vi "readFilterData.vi"() -> ()   [LabVIEW 2026]
uses:
  <vilib>/Utility/miscctls.llb/LVRectTypeDef.ctl
  <vilib>/Utility/miscctls.llb/LVPointTypeDef.ctl
  <userlib>/Sensor.ctl
  <vilib>/measure/maspectr.llb/FFT Spectrum (Mag-Phase) for N Chan.vi
  <vilib>/Analysis/3filter.llb/Butterworth Filter (DBL).vi
  <vilib>/Instr/_visa.llb/VISA Configure Serial Port (Instr).vi
  <vilib>/measure/NI_MAPro.lvlib
  <vilib>/Analysis/NI_AALBase.lvlib
panel:
  in  "Time Target (s)":dbl=60.0
  out "SyncStop 2":bool
  out "Result":dbl
  in  "UvodniStranka":bool
  in  "ExitApp":bool
  in  "error in (no error)":errorcluster
  in  "Tab Control":T1(tab)
  in  "Playground":bool
  in  "UlohaACC":bool
  in  "UlohaEDA":bool
  in  "UlohaEEG":bool
  in  "UlohaEMG":bool
  in  "UlohaEKG":bool
  in  "StartMeasureEKG":bool
  in  "StopMeasureEKG":bool
  in  "HintEKG":bool
  out "GraphEKG":waveform(dbl)[](graph)
  out "ChartEKG":dbl(graph)
  in  "Vstupní COM port 2":refnum<visa-resource-name>
  out "BPM":i32
  out "size(s)":i32
  in  "Doba mìøení (s)":dbl=1.0 caption="Time Target (s)"
  out "SpectrumPlayground":cluster{"f0":dbl, "df":dbl, "magnitude":dbl[]}[](graph)
  in  "Filtr":bool
  in  "SaveFileButton":bool
  out "Waveform Graph":waveform(dbl)[](graph)
  in  "Horní mezní frekvence":dbl=0.45000000000000007 format="%0.2f"
  in  "Dolní mezní frekvence":dbl=0.12500000000000006 format="%0.4f"
  in  "Typ filtru":T2(ring)
  in  "OdstranitFiltr":bool
  in  "DeleteSignal":bool
  out "Waveform Chart":dbl(graph)
  in  "SendToFilter":bool
  out "Waveform":waveform(dbl)(graph)
  out "SyncStop":bool
  in  "Vstupní COM port":refnum<visa-resource-name>
  in  "Vzorkovací frekvence (Hz)":enum16{"1", "10", "100", "1000"}(ring)
  in  "Druh signálu":T3
  in  "StartMeasure":bool
  in  "StopMeasure":bool
  in  "Radio Buttons":T4(radio)
  # "Aplikace pro mìøení na platformì PLUX BITalino"
  # "EKG"
  # "Vstupní COM port"
  # "EEG"
  # "EDA"
  # "ACC"
  # "EMG"
  # "A1"
  # "A2"
  # "A3"
  # "A4"
  # "A5"
  # "A6"
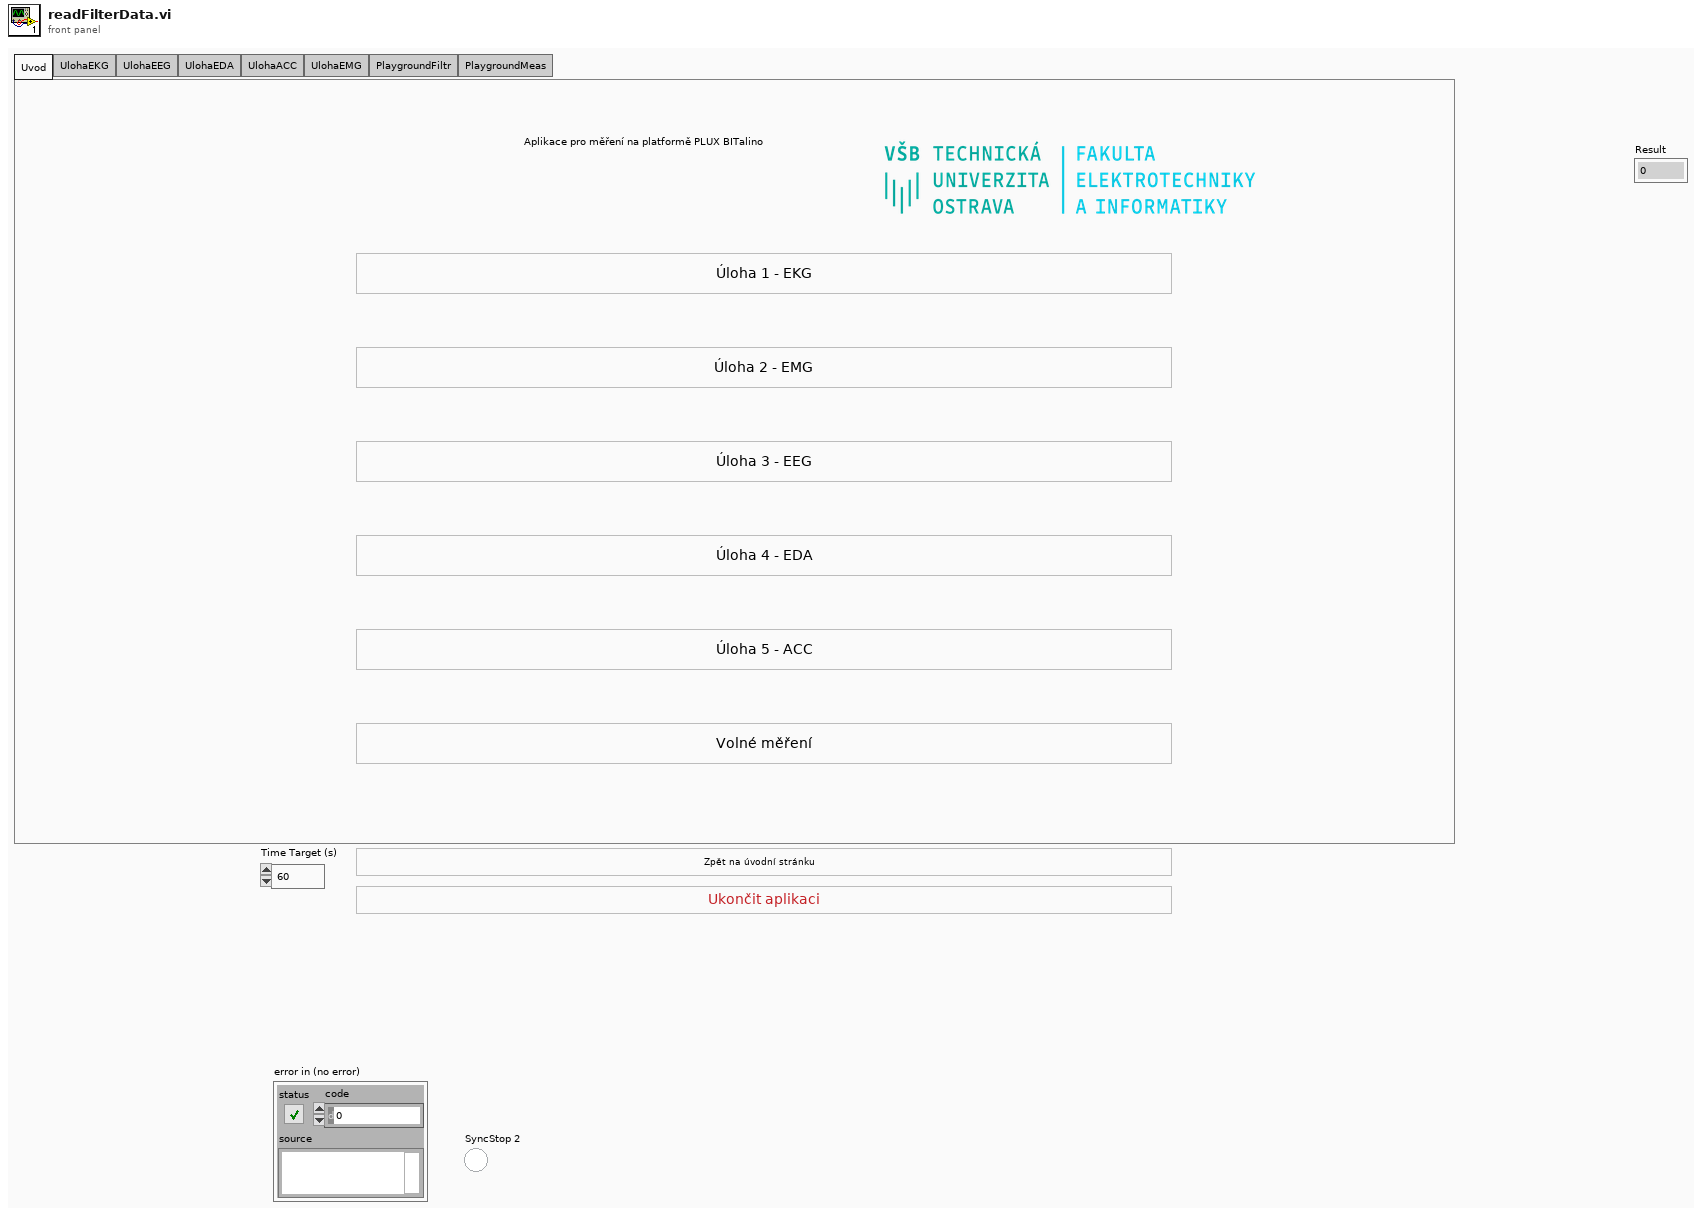
[diagram p1: front panel]
types:
  T1 = enum32{"Uvod", "UlohaEKG", "UlohaEEG", "UlohaEDA", "UlohaACC", "UlohaEMG", "PlaygroundFiltr", "PlaygroundMeas"}
  T2 = enum32{"Lowpass", "Highpass", "Bandpass", "Bandstop"}
  T3 = cluster{"Signál na kanálu A1":enum16{"EMG", "ECG", "EEG", "EDA", "ACC"}, "Signál na kanálu A2":enum16{"EMG", "ECG", "EEG", "EDA", "ACC"}, "Signál na kanálu A3":enum16{"EMG", "ECG", "EEG", "EDA", "ACC"}, "Signál na kanálu A4":enum16{"EMG", "ECG", "EEG", "EDA", "ACC"}, "Signál na kanálu A5":enum16{"EMG", "ECG", "EEG", "EDA", "ACC"}, "Signál na kanálu A6":enum16{"EMG", "ECG", "EEG", "EDA", "ACC"}}
  T4 = enum32{"Item 0", "Item 1", "Item 2", "Item 3", "Item 4", "Item 5"}
  T5 = enum16{"Wait", "Exit", "Measure", "Intro", "UlohaEKG", "UlohaEMG", "PlaygroundMeas", "UlohaEEG", "UlohaEDA", "UlohaACC", "PlaygroundFiltr", "SaveFile", "FilterSignal", "RemoveFilter", "HintEKG", "DeleteSignal"}
  T6 = enum16{"Always On", "Always Off", "Off While Running"}
  T7 = enum32{"Uvod", "UlohaEKG", "UlohaEEG", "UlohaEDA", "UlohaACC", "UlohaEMG", "PlaygroundFiltr"}
  T8 = typedef "LVPointTypeDef.ctl" = cluster{"Horizontal":i16, "Vertical":i16}
  T9 = typedef "LVRectTypeDef.ctl" = cluster{"Left":i16, "Top":i16, "Right":i16, "Bottom":i16}
  T10 = enum8{"Enabled", "Disabled", "Disabled and Grayed Out"}
  T11 = typedef "Sensor.ctl" = enum16{"EMG", "ECG", "EEG", "EDA", "ACC", "LUX"}
  T12 = cluster{"Sensor 1":T11, "Sensor 2":T11, "Sensor 3":T11, "Sensor 4":T11, "Sensor 5":T11, "Sensor 6":T11}
  T13 = cluster{"Result":dbl, "Result":dbl, "Result":dbl, "Result":dbl, "Result":dbl, "Result":dbl}
  T14 = enum16{"Wait", "Exit", "Measure", "Intro", "UlohaEKG", "UlohaEMG", "PlaygroundMeas", "UlohaEEG", "UlohaEDA", "UlohaACC", "PlaygroundFiltr", "SaveFile", "FilterSignal", "RemoveFilter", "HintEKG"}
  T15 = enum16{"Wait", "Exit", "Measure", "Intro", "UlohaEKG", "UlohaEMG", "PlaygroundMeas", "UlohaEEG", "UlohaEDA", "UlohaACC"}
  T16 = enum16{"Wait", "Exit", "Measure", "Intro", "UlohaEKG", "UlohaEMG", "PlaygroundMeas"}
  T17 = enum16{"Wait", "Exit", "Measure", "Intro", "UlohaEKG", "UlohaEMG"}
  T18 = enum16{"Wait", "Exit", "Measure", "Intro", "UlohaEKG", "UlohaEMG", "PlaygroundMeas", "UlohaEEG", "UlohaEDA", "UlohaACC", "PlaygroundFiltr"}
  T19 = enum16{"Wait", "Exit", "Measure", "Intro", "UlohaEKG", "UlohaEMG", "PlaygroundMeas", "UlohaEEG", "UlohaEDA", "UlohaACC", "PlaygroundFiltr", "SaveFile"}
  T20 = enum16{"Wait", "Exit", "Measure", "Intro", "UlohaEKG", "UlohaEMG", "PlaygroundMeas", "UlohaEEG", "UlohaEDA", "UlohaACC", "PlaygroundFiltr", "SaveFile", "FilterSignal", "RemoveFilter"}
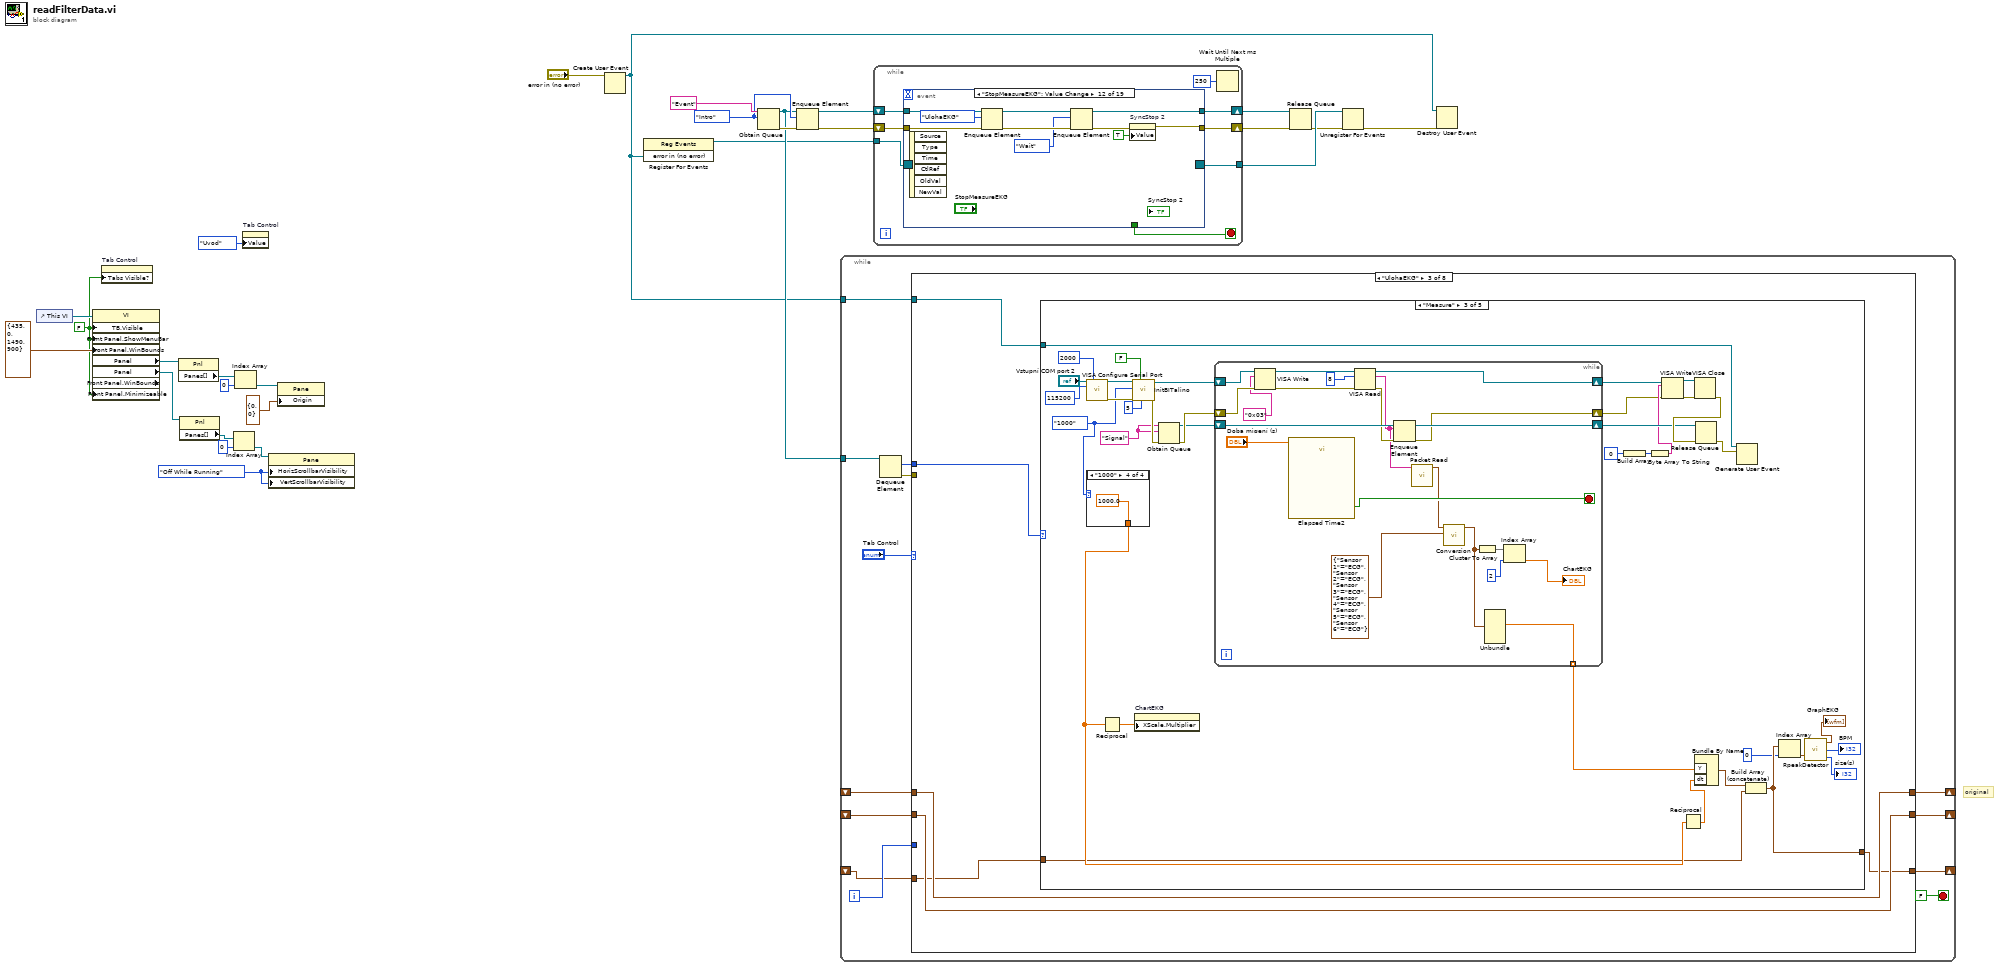
[diagram p0: block diagram]
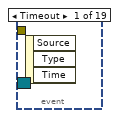
[diagram p2: hidden frame]
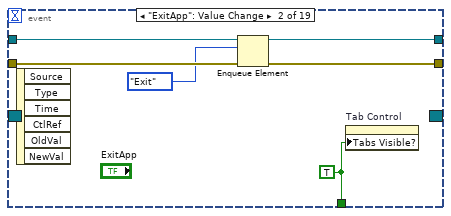
[diagram p3: hidden frame]
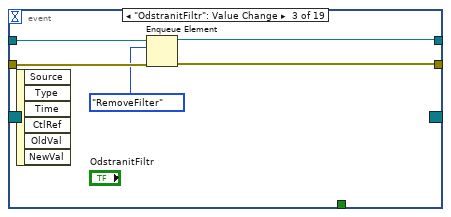
[diagram p4: hidden frame]
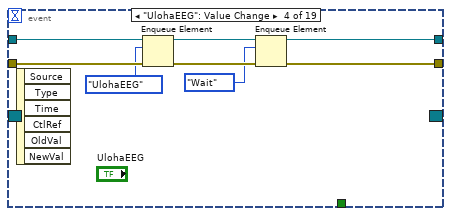
[diagram p5: hidden frame]
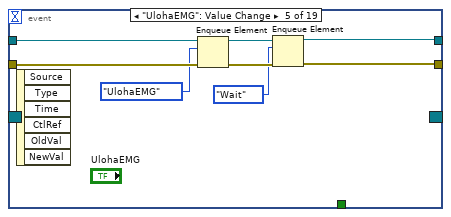
[diagram p6: hidden frame]
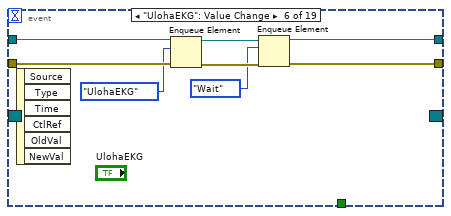
[diagram p7: hidden frame]
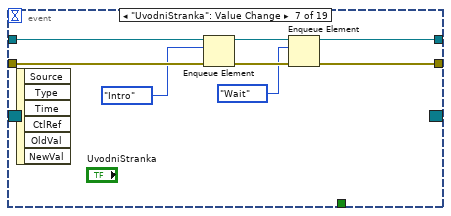
[diagram p8: hidden frame]
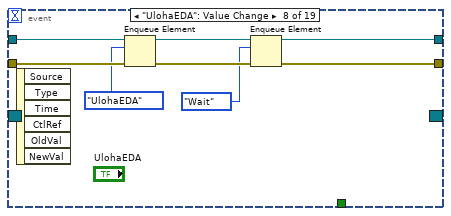
[diagram p9: hidden frame]
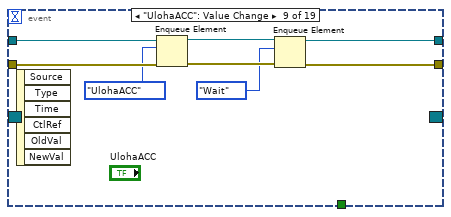
[diagram p10: hidden frame]
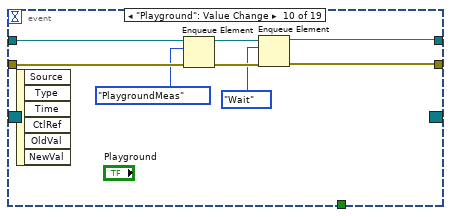
[diagram p11: hidden frame]
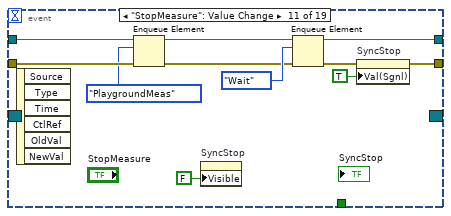
[diagram p12: hidden frame]
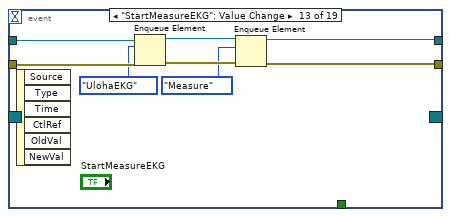
[diagram p13: hidden frame]
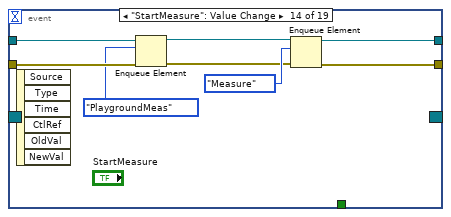
[diagram p14: hidden frame]
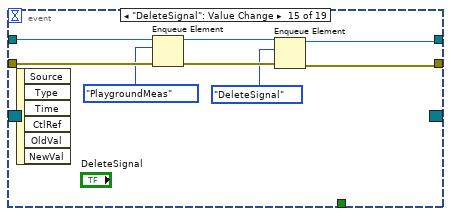
[diagram p15: hidden frame]
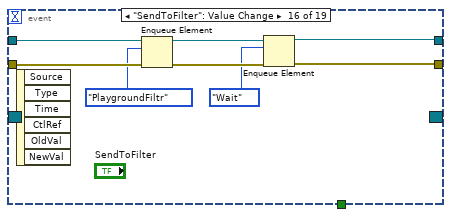
[diagram p16: hidden frame]
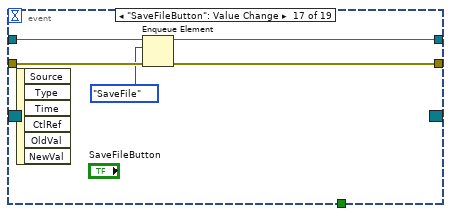
[diagram p17: hidden frame]
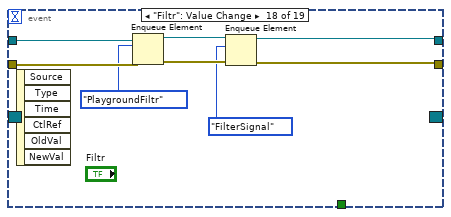
[diagram p18: hidden frame]
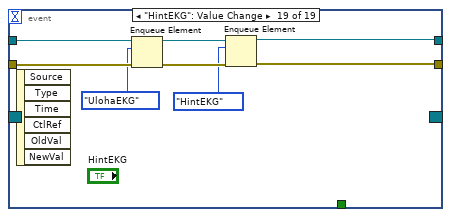
[diagram p19: hidden frame]
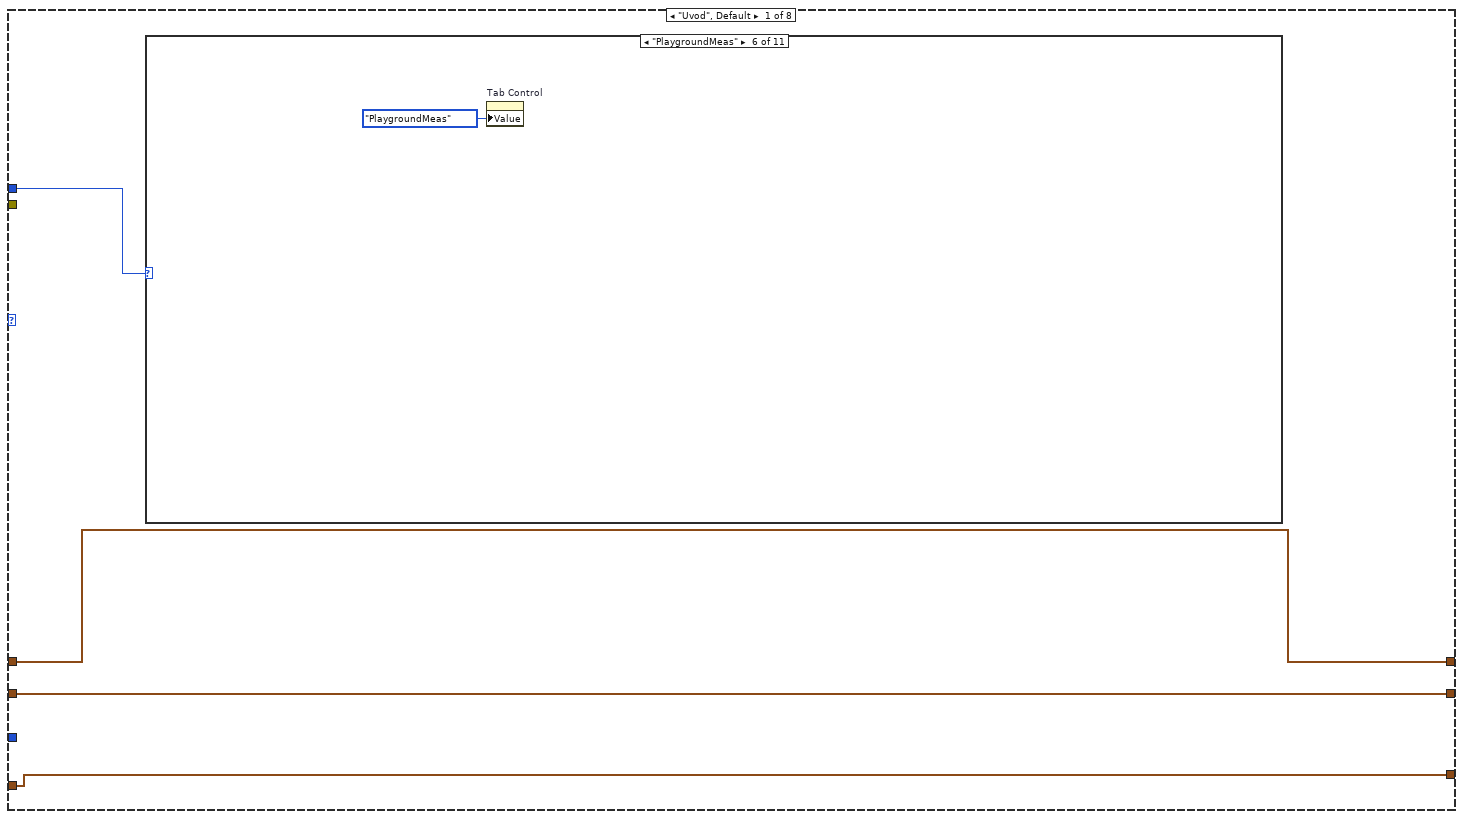
[diagram p20: hidden frame]
diagram:
  w10 = T5."Intro"
  w16 = T6."Off While Running" ("Horizontal Scrollbar Visibility")
  w15 = FALSE ("Front Panel Window:Closeable")
  # "original"
  n1 = control-ref of="This VI"() -> (w28:refnum<vi>)
  n2 = property class="VI" props=["TB.Visible", "Front Panel.ShowMenuBar", "Front Panel.WinBounds", "Panel", "Panel", "Front Panel.WinBounds", "Front Panel.Minimizeable"](reference=w28, "TB.Visible"=w15, "Front Panel.ShowMenuBar"=w15, "Front Panel.WinBounds"=T9 {"Left"=435, "Top"=0, "Right"=1490, "Bottom"=900} ("Front Panel Window:Window Bounds"), "Front Panel.Minimizeable"=w15) -> ("Panel"=w26:refnum<vi>, "Panel"=w20:refnum<vi>)  [unwired: 1 in, 3 out]
  n3 = property on="Tab Control" class="TabCtl (strict)"("Tabs Visible?"=w15) -> ()  [unwired: 2 in, 2 out]
  n4 = property class="Pnl"(reference=w26) -> ("Panes[]"=w25:refnum<vi>[])  [unwired: 1 in, 2 out]
  n5 = property class="Pnl"(reference=w20) -> ("Panes[]"=w19:refnum<vi>[])  [unwired: 1 in, 2 out]
  n6 = Index Array(array=w19, index=0) -> (element=w17:refnum<vi>)
  n7 = Index Array(array=w25, index=0) -> (element=w23:refnum<vi>)
  n8 = property on="Tab Control" class="TabCtl (strict)"("Value"=T7."Uvod" ("Tab Control")) -> ()  [unwired: 2 in, 2 out]
  n9 = property class="Pane"(reference=w17, "HorizScrollbarVisibility"=w16, "VertScrollbarVisibility"=w16) -> ()  [unwired: 1 in, 2 out]
  n10 = property class="Pane"(reference=w23, "Origin"=T8 {"Horizontal"=0, "Vertical"=0}) -> ()  [unwired: 1 in, 2 out]
  n11 = Create User Event(user event datatype="error in (no error)") -> (user event=w2:refnum<user-event>)  [unwired: 1 in, 1 out]
  n12 = register-events(w2) -> (reference out=w1:refnum<event-registration>)  [unwired: 2 in, 1 out]
  n13 = Obtain Queue(name (unnamed)="Event", element data type=w10) -> (queue out=w9:refnum<queue>, error out=w13:errorcluster)  [unwired: 3 in, 1 out]
  n14 = Enqueue Element(queue=w9, element=w10, error in (no error)=w13) -> (queue out=w12:refnum<queue>, error out=w11:errorcluster)  [unwired: 1 in, 1 out]
  n15 = while {
    shift-right: [w41] -> _
    shift-left: _ -> [w33]
    tunnel: w9 -> [w37]
    tunnel: w2 -> [w36]
    shift-right: [w32] -> _
    shift-left: _ -> [w31]
    shift-right: [w30] -> _
    shift-left: _ -> [w29]
    i -> [w40]
    stop <- FALSE stop-if-true
    n16 = Dequeue Element(queue=w37) -> (element=w38:T5, error out=w35:errorcluster)  [unwired: 2 in, 2 out]
    n17 = case shown="\"UlohaEKG\"" "Tab Control" {
      tunnel: [w45 w60 w96 w172 w180 w188 w196 w204] -> w41
      tunnel: w33 -> [w45 w61 w96 w172 w180 w188 w196 w203]
      tunnel: w40 -> [_ _ _ _ _ _ _ _]
      tunnel: w38 -> [w44 w62 w99 w171 w179 w187 w195 w207]
      tunnel: w36 -> [_ _ w98 _ _ _ _ w206]
      tunnel: w35 -> [_ _ _ _ _ _ _ w205]
      tunnel: [w43 w59 w97 w170 w178 w186 w194 w202] -> w32
      tunnel: w31 -> [w43 w58 w97 w170 w178 w186 w194 w202]
      tunnel: [w42 w57 w95 w169 w177 w185 w193 w201] -> w30
      tunnel: w29 -> [w42 w57 w94 w169 w177 w185 w193 w201]
      frame "Uvod", Default {
        n18 = case shown="\"PlaygroundMeas\"" w44 {
          frame "Wait", Default {
            n19 = property on="UvodniStranka" class="Bool"("DisabledEnum"=T10."Disabled and Grayed Out" ("Disabled")) -> ()  [unwired: 2 in, 2 out]
            n20 = property on="Tab Control" class="TabCtl (strict)"("Tabs Visible?"=FALSE) -> ()  [unwired: 2 in, 2 out]
          }
          frame "UlohaEKG" {
            n21 = property on="Tab Control" class="TabCtl (strict)"("Value"=T1."UlohaEKG" ("Tab Control")) -> ()  [unwired: 2 in, 2 out]
          }
          frame "UlohaEMG" {
            n22 = property on="Tab Control" class="TabCtl (strict)"("Value"=T1."UlohaEMG" ("Tab Control")) -> ()  [unwired: 2 in, 2 out]
          }
          frame "Exit" {
            n23 = flat-sequence {
              frame #0 {
                n24 = property on="Tab Control" class="TabCtl (strict)"("Value"=T1."Uvod" ("Tab Control")) -> ()  [unwired: 2 in, 2 out]
              }
              frame #1 {
                n25 = Stop(stop? (T)=TRUE) -> ()
              }
            }
          }
          frame "Intro" {
            n26 = property on="Tab Control" class="TabCtl (strict)"("Value"=T1."Uvod" ("Tab Control")) -> ()  [unwired: 2 in, 2 out]
          }
          frame "PlaygroundMeas" {
            n27 = property on="Tab Control" class="TabCtl (strict)"("Value"=T1."PlaygroundMeas" ("Tab Control")) -> ()  [unwired: 2 in, 2 out]
          }
          frame "Measure" {
          }
          frame "UlohaEEG" {
            n28 = property on="Tab Control" class="TabCtl (strict)"("Value"=T1."UlohaEEG" ("Tab Control")) -> ()  [unwired: 2 in, 2 out]
          }
          frame "UlohaEDA" {
            n29 = property on="Tab Control" class="TabCtl (strict)"("Value"=T1."UlohaEDA" ("Tab Control")) -> ()  [unwired: 2 in, 2 out]
          }
          frame "UlohaACC" {
            n30 = property on="Tab Control" class="TabCtl (strict)"("Value"=T1."UlohaACC" ("Tab Control")) -> ()  [unwired: 2 in, 2 out]
          }
          frame "PlaygroundFiltr" {
          }
        }
      }
      frame "PlaygroundFiltr" {
        n31 = case shown="\"RemoveFilter\"" w62 {
          tunnel: w61 -> [w64 w71 w82 w84 w88 w92]
          tunnel: [w64 w69 w82 w84 w88 w92] -> w60
          tunnel: [w64 w69 w79 w83 w87 w91] -> w59
          tunnel: w58 -> [_ w68 w79 w83 w87 w91]
          frame "Wait", Default {
            n32 = property on="UvodniStranka" class="Bool"("DisabledEnum"=T10."Enabled" ("Disabled")) -> ()  [unwired: 2 in, 2 out]
            n33 = Build Array(w64) -> (w63:waveform(dbl)[])
            "Waveform Graph" <- w63
            n34 = call-poly <vilib>:"FFT Spectrum (Mag-Phase).vi"("time signals"=w63) -> ("magnitudes"=w65:cluster{"f0":dbl, "df":dbl, "magnitude":dbl[]}[])  [unwired: 6 in, 4 out]
            n35 = local write "SpectrumPlayground"(w65) -> ()
          }
          frame "FilterSignal" {
            n36 = Unbundle By Name(w71) -> ("Y"=w73:dbl[], "dt"=w70:dbl)
            n37 = Reciprocal(x=w70) -> (1/x=w72:dbl)
            n38 = call-poly <vilib>:"Butterworth Filter.vi"("filter type"="Typ filtru", "low cutoff freq: fl"="Dolní mezní frekvence", "high cutoff freq: fh"="Horní mezní frekvence", "sampling freq: fs"=w72, "X"=w73) -> ("Filtered X"=w74:dbl[])  [unwired: 3 in, 1 out]
            n39 = Bundle By Name("Y"=w74, "dt"=w70) -> (w69:waveform(dbl))  [unwired: 1 in]
            n40 = Build Array(w68, w69) -> (w67:waveform(dbl)[])
            n41 = call-poly <vilib>:"FFT Spectrum (Mag-Phase).vi"("time signals"=w67) -> ("magnitudes"=→"SpectrumPlayground":cluster{"f0":dbl, "df":dbl, "magnitude":dbl[]}[])  [unwired: 6 in, 4 out]
            n42 = local write "Waveform Graph"(w67) -> ()
          }
          frame "RemoveFilter" {
            n43 = Build Array(w79, w79) -> (w80:waveform(dbl)[])
            n44 = local write "Waveform Graph"(w80) -> ()
            n45 = call-poly <vilib>:"FFT Spectrum (Mag-Phase).vi"("time signals"=w80) -> ("magnitudes"=w81:cluster{"f0":dbl, "df":dbl, "magnitude":dbl[]}[])  [unwired: 6 in, 4 out]
            n46 = local write "SpectrumPlayground"(w81) -> ()
          }
          frame "Exit" {
            n47 = flat-sequence {
              frame #0 {
                n48 = property on="Tab Control" class="TabCtl (strict)"("Value"=T1."Uvod" ("Tab Control")) -> ()  [unwired: 2 in, 2 out]
              }
              frame #1 {
                n49 = Stop(stop? (T)=TRUE) -> ()
              }
            }
          }
          frame "Intro" {
            n50 = property on="Tab Control" class="TabCtl (strict)"("Value"=T1."Uvod" ("Tab Control")) -> ()  [unwired: 2 in, 2 out]
          }
          frame "SaveFile" {
            n51 = local read "Waveform"() -> (w93:waveform(dbl))
            n52 = call "saveFile(subVI).vi"("Typ signálu"="EMG", "Vstupní signál"=w93) -> ()  [unwired: 1 in]
          }
        }
      }
      frame "UlohaEKG" {
        n53 = case shown="\"Measure\"" w99 {
          tunnel: w98 -> [_ _ w120 _ _]
          tunnel: [w100 w102 w112 w166 w167] -> w95
          tunnel: w94 -> [w100 w102 w113 w166 w167]
          frame "Wait", Default {
            n54 = property on="UvodniStranka" class="Bool"("DisabledEnum"=T10."Enabled" ("Disabled")) -> ()  [unwired: 2 in, 2 out]
          }
          frame "Exit" {
            n55 = flat-sequence {
              frame #0 {
                n56 = property on="Tab Control" class="TabCtl (strict)"("Value"=T1."Uvod" ("Tab Control")) -> ()  [unwired: 2 in, 2 out]
              }
              frame #1 {
                n57 = Stop(stop? (T)=TRUE) -> ()
              }
            }
          }
          frame "Measure" {
            w115 = enum16{"1", "10", "100", "1000"}."1000" ("Sample Rate")
            w122 = "Signal" ("name (unnamed)")
            n58 = call-poly "VISA Configure Serial Port"("VISA resource name"="Vstupní COM port 2", "timeout (10sec)"=u32 2000, "baud rate (9600)"=u32 115200) -> ("VISA resource name out"=w137:refnum<visa-resource-name>, "error out"=w136:errorcluster)  [unwired: 11 in]
            n59 = case shown="\"1000\"" w115 {
              tunnel: [1.0 10.0 100.0 1000.0] -> w116
              frame "1", Default {
              }
              frame "10" {
              }
              frame "100" {
              }
              frame "1000" {
              }
            }
            n60 = Reciprocal(x=w116) -> (1/x=w117:dbl)
            n61 = call "InitBITalino.vi"("Battery \nThreshold (%)"=u8 5 ("Battery \nThreshold (%)"), "MODE"=FALSE, "error in (no error)"=w136, "Sample Rate"=w115, "BITalino"=w137) -> ("error out"=w132:errorcluster, "VISA out"=w133:refnum<visa-resource-name>)  [unwired: 4 in, 1 out]
            n62 = property on="ChartEKG" class="WFChart (strict)"("XScale.Multiplier"=w117) -> ()  [unwired: 2 in, 2 out]
            n63 = Obtain Queue(name (unnamed)=w122, element data type=w122, error in (no error)=w132) -> (queue out=w119:refnum<queue>, error out=w131:errorcluster)  [unwired: 2 in, 1 out]
            n64 = while {
              shift-right: [w161] -> w130
              shift-left: w133 -> [w165]
              shift-right: [w157] -> w106
              shift-left: w131 -> [w164]
              shift-right: [w158] -> w126
              shift-left: w119 -> [w160]
              tunnel: [w146] -> w105 mode=indexing
              stop <- w156 stop-if-true
              n65 = VISA Write(VISA resource name=w165, write buffer="0x03", error in (no error)=w164) -> (VISA resource name out=w154:refnum<visa-resource-name>, error out=w162:errorcluster)  [unwired: 1 out]
              n66 = call "Elapsed Time2"("Time Target (s)"="Doba mìøení (s)") -> ("Time has Elapsed"=w156:bool)  [unwired: 11 in, 7 out]
              n67 = VISA Read(VISA resource name=w154, byte count=u32 8, error in (no error)=w162) -> (VISA resource name out=w161:refnum<visa-resource-name>, read buffer=w145:string, error out=w159:errorcluster)  [unwired: 1 out]
              n68 = Enqueue Element(queue=w160, element=w145, error in (no error)=w159) -> (queue out=w158:refnum<queue>, error out=w157:errorcluster)  [unwired: 1 in, 1 out]
              n69 = call "Packet Read.vi"("Packets"=w145) -> ("Analog Channels"=w147:cluster{u16, u16, u16, u16, u16, u16})  [unwired: 7 in, 3 out]
              n70 = call "Conversion.vi"("Sensor Type"=T12 {"Sensor 1"=enum."ECG", "Sensor 2"=enum."ECG", "Sensor 3"=enum."ECG", "Sensor 4"=enum."ECG", "Sensor 5"=enum."ECG", "Sensor 6"=enum."ECG"}, "Analog Channels"=w147) -> ("output cluster"=w148:T13)  [unwired: 8 in, 1 out]
              n71 = Cluster To Array(cluster=w148) -> (array=w151:dbl[])
              n72 = Unbundle(w148) -> ("Result"=w146:dbl)  [unwired: 5 out]
              n73 = Index Array(array=w151, index=2) -> (element=→"ChartEKG":dbl)
            }
            n74 = Build Array(u8 0) -> (w124:u8[])
            n75 = Byte Array To String(unsigned byte array=w124) -> (string=w123:string)
            n76 = VISA Write(VISA resource name=w130, write buffer=w123, error in (no error)=w106) -> (VISA resource name out=w129:refnum<visa-resource-name>, error out=w128:errorcluster)  [unwired: 1 out]
            n77 = Reciprocal(x=w116) -> (1/x=w118:dbl)
            n78 = VISA Close(VISA resource name=w129, error in (no error)=w128) -> (error out=w127:errorcluster)
            n79 = Bundle By Name("Y"=w105, "dt"=w118) -> (w114:waveform(dbl))  [unwired: 1 in]
            n80 = Release Queue(queue=w126, error in (no error)=w127) -> (error out=w121:errorcluster)  [unwired: 1 in, 2 out]
            n81 = Generate User Event(user event=w120, event data cluster=w121) -> ()  [unwired: 2 in, 2 out]
            n82 = Build Array (concatenate)(w114, w113) -> (w112:waveform(dbl)[])
            n83 = Index Array(array=w112, index=0) -> (element=w110:waveform(dbl))
            n84 = call "RpeakDetector.vi"("Vstupní signál"=w110) -> ("Signál s peaky"=→"GraphEKG":waveform(dbl)[], "BPM"=→"BPM":i32, "size(s)"=→"size(s)":i32)
          }
          frame "HintEKG" {
            n85 = call "NapovedaEKG(subVI).vi"() -> ()  [unwired: 1 in]
          }
          frame "Intro" {
            n86 = property on="Tab Control" class="TabCtl (strict)"("Value"=T1."Uvod" ("Tab Control")) -> ()  [unwired: 2 in, 2 out]
          }
        }
      }
      frame "UlohaEEG" {
        n87 = case shown="\"Exit\"" w171 {
          frame "Wait", Default {
            n88 = property on="UvodniStranka" class="Bool"("DisabledEnum"=T10."Enabled" ("Disabled")) -> ()  [unwired: 2 in, 2 out]
          }
          frame "Exit" {
            n89 = flat-sequence {
              frame #0 {
                n90 = property on="Tab Control" class="TabCtl (strict)"("Value"=T1."Uvod" ("Tab Control")) -> ()  [unwired: 2 in, 2 out]
              }
              frame #1 {
                n91 = Stop(stop? (T)=TRUE) -> ()
              }
            }
          }
          frame "Measure" {
          }
          frame "Intro" {
            n92 = property on="Tab Control" class="TabCtl (strict)"("Value"=T1."Uvod" ("Tab Control")) -> ()  [unwired: 2 in, 2 out]
          }
          frame "UlohaEKG" {
          }
          frame "UlohaEMG" {
          }
          frame "PlaygroundMeas" {
          }
          frame "UlohaEEG" {
          }
          frame "UlohaEDA" {
          }
          frame "UlohaACC" {
          }
        }
      }
      frame "UlohaEDA" {
        n93 = case shown="\"Wait\", Default" w179 {
          frame "Wait", Default {
            n94 = property on="UvodniStranka" class="Bool"("DisabledEnum"=T10."Enabled" ("Disabled")) -> ()  [unwired: 2 in, 2 out]
          }
          frame "Exit" {
            n95 = flat-sequence {
              frame #0 {
                n96 = property on="Tab Control" class="TabCtl (strict)"("Value"=T1."Uvod" ("Tab Control")) -> ()  [unwired: 2 in, 2 out]
              }
              frame #1 {
                n97 = Stop(stop? (T)=TRUE) -> ()
              }
            }
          }
          frame "Measure" {
          }
          frame "Intro" {
            n98 = property on="Tab Control" class="TabCtl (strict)"("Value"=T1."Uvod" ("Tab Control")) -> ()  [unwired: 2 in, 2 out]
          }
          frame "UlohaEKG" {
          }
          frame "UlohaEMG" {
          }
          frame "PlaygroundMeas" {
          }
          frame "UlohaEEG" {
          }
          frame "UlohaEDA" {
          }
          frame "UlohaACC" {
          }
        }
      }
      frame "UlohaACC" {
        n99 = case shown="\"Wait\", Default" w187 {
          frame "Wait", Default {
            n100 = property on="UvodniStranka" class="Bool"("DisabledEnum"=T10."Enabled" ("Disabled")) -> ()  [unwired: 2 in, 2 out]
          }
          frame "Exit" {
            n101 = flat-sequence {
              frame #0 {
                n102 = property on="Tab Control" class="TabCtl (strict)"("Value"=T1."Uvod" ("Tab Control")) -> ()  [unwired: 2 in, 2 out]
              }
              frame #1 {
                n103 = Stop(stop? (T)=TRUE) -> ()
              }
            }
          }
          frame "Measure" {
          }
          frame "Intro" {
            n104 = property on="Tab Control" class="TabCtl (strict)"("Value"=T1."Uvod" ("Tab Control")) -> ()  [unwired: 2 in, 2 out]
          }
          frame "UlohaEKG" {
          }
          frame "UlohaEMG" {
          }
          frame "PlaygroundMeas" {
          }
          frame "UlohaEEG" {
          }
          frame "UlohaEDA" {
          }
          frame "UlohaACC" {
          }
        }
      }
      frame "UlohaEMG" {
        n105 = case shown="\"Intro\"" w195 {
          frame "Wait", Default {
            n106 = property on="UvodniStranka" class="Bool"("DisabledEnum"=T10."Enabled" ("Disabled")) -> ()  [unwired: 2 in, 2 out]
          }
          frame "Exit" {
            n107 = flat-sequence {
              frame #0 {
                n108 = property on="Tab Control" class="TabCtl (strict)"("Value"=T1."Uvod" ("Tab Control")) -> ()  [unwired: 2 in, 2 out]
              }
              frame #1 {
                n109 = Stop(stop? (T)=TRUE) -> ()
              }
            }
          }
          frame "Measure" {
          }
          frame "Intro" {
            n110 = property on="Tab Control" class="TabCtl (strict)"("Value"=T1."Uvod" ("Tab Control")) -> ()  [unwired: 2 in, 2 out]
          }
          frame "UlohaEKG" {
          }
          frame "UlohaEMG" {
          }
          frame "PlaygroundMeas" {
          }
        }
      }
      frame "PlaygroundMeas" {
        n111 = case shown="No Error" w205 {
          tunnel: w207 -> [w212 _]
          tunnel: [FALSE TRUE] -> _
          tunnel: w206 -> [w210 _]
          tunnel: [w209 w320] -> w204
          tunnel: w203 -> [w208 w320]
          frame No Error {
            n112 = case shown="\"Measure\"" w212 {
              tunnel: w210 -> [_ _ _ _ w236 _]
              tunnel: [w213 w216 w222 w224 w228 w317] -> w209
              tunnel: w208 -> [w213 w216 w222 w224 _ w317]
              frame "Wait", Default {
                n113 = property on="UvodniStranka" class="Bool"("DisabledEnum"=T10."Enabled" ("Disabled")) -> ()  [unwired: 2 in, 2 out]
                n114 = property on="SyncStop" class="Bool (strict)"("Val(Sgnl)"=FALSE ("Value (Signaling)")) -> ()  [unwired: 2 in, 2 out]
              }
              frame "Exit" {
                n115 = flat-sequence {
                  frame #0 {
                    w218 = waveform(dbl) {"t0"=timestamp(0 s since 1904-01-01), "dt"=1.0, "Y"=[0.0]} ("Waveform")
                    n116 = property on="Tab Control" class="TabCtl (strict)"("Value"=T1."Uvod" ("Tab Control")) -> ()  [unwired: 2 in, 2 out]
                    n117 = Build Array(w218, w218) -> (w217:waveform(dbl)[])
                    n118 = call-poly <vilib>:"FFT Spectrum (Mag-Phase).vi"("time signals"=w217) -> ("magnitudes"=w219:cluster{"f0":dbl, "df":dbl, "magnitude":dbl[]}[])  [unwired: 6 in, 4 out]
                    n119 = local write "SpectrumPlayground"(w219) -> ()
                    n120 = property on="Waveform Graph" class="WFGraph (strict)"("Value"=w217) -> ()  [unwired: 2 in, 2 out]
                  }
                  frame #1 {
                    n121 = Stop(stop? (T)=TRUE) -> ()
                  }
                }
              }
              frame "PlaygroundFiltr" {
                n122 = property on="Tab Control" class="TabCtl (strict)"("Value"=T1."PlaygroundFiltr" ("Tab Control")) -> ()  [unwired: 2 in, 2 out]
              }
              frame "Intro" {
                n123 = flat-sequence {
                  frame #0 {
                    n124 = property on="Tab Control" class="TabCtl (strict)"("Value"=T1."Uvod" ("Tab Control")) -> ()  [unwired: 2 in, 2 out]
                  }
                  frame #1 {
                    n125 = Wait (ms)(milliseconds to wait=u32 100) -> ()  [unwired: 1 out]
                  }
                }
              }
              frame "Measure" {
                w238 = "Signal" ("name (unnamed)")
                n126 = property on="Vzorkovací frekvence (Hz)" class="Enum (strict)"() -> ("Value"=w231:enum16{"1", "10", "100", "1000"})  [unwired: 2 in, 2 out]
                n127 = call-poly "VISA Configure Serial Port"("VISA resource name"="Vstupní COM port", "timeout (10sec)"=u32 2000, "baud rate (9600)"=u32 115200) -> ("VISA resource name out"=w253:refnum<visa-resource-name>, "error out"=w252:errorcluster)  [unwired: 11 in]
                n128 = case shown="\"1000\"" w231 {
                  tunnel: [1.0 10.0 100.0 1000.0] -> w227
                  frame "1", Default {
                  }
                  frame "10" {
                  }
                  frame "100" {
                  }
                  frame "1000" {
                  }
                }
                n129 = Reciprocal(x=w227) -> (1/x=w230:dbl)
                n130 = call "InitBITalino.vi"("Battery \nThreshold (%)"=u8 5 ("Battery \nThreshold (%)"), "MODE"=FALSE, "error in (no error)"=w252, "Sample Rate"="Vzorkovací frekvence (Hz)", "BITalino"=w253) -> ("error out"=w248:errorcluster, "VISA out"=w249:refnum<visa-resource-name>)  [unwired: 4 in, 1 out]
                n131 = property on="Waveform Chart" class="WFChart (strict)"("XScale.Multiplier"=w230) -> ()  [unwired: 2 in, 2 out]
                n132 = Obtain Queue(name (unnamed)=w238, element data type=w238, error in (no error)=w248) -> (queue out=w237:refnum<queue>, error out=w247:errorcluster)  [unwired: 2 in, 1 out]
                n133 = while {
                  shift-right: [w310] -> w246
                  shift-left: w249 -> [w316]
                  shift-right: [w305] -> w229
                  shift-left: w247 -> [w315]
                  shift-right: [w306] -> w242
                  shift-left: w237 -> [w309]
                  stop <- w304 stop-if-true
                  n134 = VISA Write(VISA resource name=w316, write buffer="0x03", error in (no error)=w315) -> (VISA resource name out=w313:refnum<visa-resource-name>, error out=w312:errorcluster)  [unwired: 1 out]
                  n135 = call "Elapsed Time"("Time Target (s)"="Time Target (s)") -> ("Time has Elapsed"=w302:bool)  [unwired: 11 in, 7 out]
                  n136 = VISA Read(VISA resource name=w313, byte count=u32 8, error in (no error)=w312) -> (VISA resource name out=w310:refnum<visa-resource-name>, read buffer=w308:string, error out=w307:errorcluster)  [unwired: 1 out]
                  n137 = Enqueue Element(queue=w309, element=w308, error in (no error)=w307) -> (queue out=w306:refnum<queue>, error out=w305:errorcluster)  [unwired: 1 in, 1 out]
                  n138 = Unbundle By Name(w305) -> ("status"=w303:bool)
                  n139 = Or(x=w303, y=w302) -> (x .or. y?=w304:bool)
                }
                n140 = while {
                  tunnel: w237 -> [w266]
                  tunnel: [w262] -> w234 mode=indexing
                  tunnel: "Radio Buttons" -> [w261]
                  stop <- w263 stop-if-true
                  n141 = Dequeue Element(queue=w266) -> (element=w265:string, error out=w264:errorcluster)  [unwired: 2 in, 2 out]
                  n142 = case shown="No Error" w264 {
                    tunnel: w265 -> [w273 _]
                    tunnel: [FALSE TRUE] -> w263
                    tunnel: [w268 w299] -> w262
                    tunnel: w261 -> [w270 _]
                    frame No Error {
                      n143 = call "Packet Read.vi"("Packets"=w273) -> ("Analog Channels"=w272:cluster{u16, u16, u16, u16, u16, u16})  [unwired: 7 in, 3 out]
                      n144 = call "Conversion.vi"("Sensor Type"="Druh signálu", "Analog Channels"=w272) -> ("output cluster"=w269:T13)  [unwired: 8 in, 1 out]
                      n145 = case shown="\"Item 2\"" w270 {
                        tunnel: w269 -> [w277 w279 w284 w288 w292 w296]
                        tunnel: [w274 w278 w283 w287 w291 w295] -> w268
                        tunnel: "Druh signálu" -> [_ _ _ _ _ _]
                        frame "Item 0", Default {
                          n146 = Cluster To Array(cluster=w277) -> (array=w276:dbl[])
                          n147 = Index Array(array=w276, index=0) -> ()  [unwired: 1 out]
                          n148 = Unbundle(w277) -> ("Result"=w274:dbl)  [unwired: 5 out]
                        }
                        frame "Item 1" {
                          n149 = Cluster To Array(cluster=w279) -> (array=w281:dbl[])
                          n150 = Index Array(array=w281, index=1) -> ()  [unwired: 1 out]
                          n151 = Unbundle(w279) -> ("Result"=w278:dbl)  [unwired: 5 out]
                        }
                        frame "Item 2" {
                          n152 = Cluster To Array(cluster=w284) -> (array=w286:dbl[])
                          n153 = Unbundle(w284) -> ("Result"=w283:dbl)  [unwired: 5 out]
                          n154 = Index Array(array=w286, index=2) -> (element=→"Waveform Chart":dbl)
                        }
                        frame "Item 3" {
                          n155 = Cluster To Array(cluster=w288) -> (array=w290:dbl[])
                          n156 = Unbundle(w288) -> ("Result"=w287:dbl)  [unwired: 5 out]
                          n157 = Index Array(array=w290, index=3) -> ()  [unwired: 1 out]
                        }
                        frame "Item 4" {
                          n158 = Cluster To Array(cluster=w292) -> (array=w294:dbl[])
                          n159 = Unbundle(w292) -> ("Result"=w291:dbl)  [unwired: 5 out]
                          n160 = Index Array(array=w294, index=4) -> ()  [unwired: 1 out]
                        }
                        frame "Item 5" {
                          n161 = Cluster To Array(cluster=w296) -> (array=w298:dbl[])
                          n162 = Unbundle(w296) -> ("Result"=w295:dbl)  [unwired: 5 out]
                          n163 = Index Array(array=w298, index=5) -> ()  [unwired: 1 out]
                        }
                      }
                      "Result" <- w268
                    }
                    frame Error {
                      n164 = local read "Result"() -> (w299:dbl)
                    }
                  }
                }
                n165 = Build Array(u8 0) -> (w240:u8[])
                n166 = Byte Array To String(unsigned byte array=w240) -> (string=w239:string)
                n167 = VISA Write(VISA resource name=w246, write buffer=w239, error in (no error)=w229) -> (VISA resource name out=w245:refnum<visa-resource-name>, error out=w244:errorcluster)  [unwired: 1 out]
                n168 = VISA Close(VISA resource name=w245, error in (no error)=w244) -> (error out=w243:errorcluster)
                n169 = Release Queue(queue=w242, error in (no error)=w243) -> (error out=w235:errorcluster)  [unwired: 1 in, 2 out]
                n170 = Generate User Event(user event=w236, event data cluster=w235) -> ()  [unwired: 2 in, 2 out]
                n171 = Bundle By Name("Y"=w234, "dt"=w230) -> (w228:waveform(dbl))  [unwired: 1 in]
                "Waveform" <- w228
              }
              frame "DeleteSignal" {
                n172 = property on="Waveform Chart" class="WFChart (strict)"("History Data"=dbl[] []) -> ()  [unwired: 2 in, 2 out]
                n173 = local write "Waveform"(waveform(dbl) {"t0"=timestamp(0 s since 1904-01-01), "dt"=1.0, "Y"=[]} ("Waveform")) -> ()
              }
            }
          }
          frame Error {
          }
        }
      }
    }
  }
  n174 = while {
    shift-right: [w327] -> w7
    shift-left: w11 -> [w326]
    shift-right: [w328] -> w8
    shift-left: w12 -> [w329]
    tunnel: [w323] -> w5
    tunnel: w1 -> [w322]
    stop <- w325 stop-if-true
    n175 = event shown="[11] \"StopMeasureEKG\": Value Change" {
      selector: w322 -> [_ _ _ _ _ _ _ _ _ _ _ _ _ _ _ _ _ _ _]
      dyn-events: [_ _ _ _ _ _ _ _ _ _ _ _ _ _ _ _ _ _ _] -> w323
      timeout: _ -> [_ _ _ _ _ _ _ _ _ _ _ _ _ _ _ _ _ _ _]
      tunnel: w329 -> [_ w335 w340 w348 w356 w364 w372 w380 w388 w396 w401 w417 w425 w430 w441 w449 w454 w462 w470]
      tunnel: w326 -> [_ w334 w338 w347 w355 w363 w371 w379 w387 w395 w399 w416 w424 w428 w440 w448 w453 w459 w467]
      tunnel: [_ w333 w339 w344 w352 w360 w367 w377 w385 w390 w406 w413 w422 w433 w437 w445 w452 w460 w468] -> w328
      tunnel: [_ w332 w337 w342 w351 w358 w366 w376 w383 w392 w403 w409 w420 w432 w435 w443 w451 w457 w465] -> w327
      tunnel: [_ w330 _ _ _ _ _ _ _ _ _ _ _ _ _ _ _ _ _] -> w325
      event Timeout {
        n176 = event-data() -> ()  [unwired: 1 in, 3 out]
      }
      event "ExitApp": Value Change {
        w330 = TRUE
        n177 = event-data() -> ()  [unwired: 1 in, 6 out]
        n178 = Enqueue Element(queue=w335, element=enum16{"Wait", "Exit", "Measure"}."Exit", error in (no error)=w334) -> (queue out=w333:refnum<queue>, error out=w332:errorcluster)  [unwired: 1 in, 1 out]
        n179 = property on="Tab Control" class="TabCtl (strict)"("Tabs Visible?"=w330) -> ()  [unwired: 2 in, 2 out]
      }
      event "OdstranitFiltr": Value Change {
        n180 = event-data() -> ()  [unwired: 1 in, 6 out]
        n181 = Enqueue Element(queue=w340, element=T14."RemoveFilter", error in (no error)=w338) -> (queue out=w339:refnum<queue>, error out=w337:errorcluster)  [unwired: 1 in, 1 out]
      }
      event "UlohaEEG": Value Change {
        n182 = event-data() -> ()  [unwired: 1 in, 6 out]
        n183 = Enqueue Element(queue=w348, element=T15."UlohaEEG", error in (no error)=w347) -> (queue out=w345:refnum<queue>, error out=w343:errorcluster)  [unwired: 1 in, 1 out]
        n184 = Enqueue Element(queue=w345, element=T15."Wait", error in (no error)=w343) -> (queue out=w344:refnum<queue>, error out=w342:errorcluster)  [unwired: 1 in, 1 out]
      }
      event "UlohaEMG": Value Change {
        n185 = event-data() -> ()  [unwired: 1 in, 6 out]
        n186 = Enqueue Element(queue=w356, element=T16."UlohaEMG", error in (no error)=w355) -> (queue out=w353:refnum<queue>, error out=w350:errorcluster)  [unwired: 1 in, 1 out]
        n187 = Enqueue Element(queue=w353, element=T16."Wait", error in (no error)=w350) -> (queue out=w352:refnum<queue>, error out=w351:errorcluster)  [unwired: 1 in, 1 out]
      }
      event "UlohaEKG": Value Change {
        n188 = event-data() -> ()  [unwired: 1 in, 6 out]
        n189 = Enqueue Element(queue=w364, element=T17."UlohaEKG", error in (no error)=w363) -> (queue out=w361:refnum<queue>, error out=w359:errorcluster)  [unwired: 1 in, 1 out]
        n190 = Enqueue Element(queue=w361, element=T17."Wait", error in (no error)=w359) -> (queue out=w360:refnum<queue>, error out=w358:errorcluster)  [unwired: 1 in, 1 out]
      }
      event "UvodniStranka": Value Change {
        n191 = event-data() -> ()  [unwired: 1 in, 6 out]
        n192 = Enqueue Element(queue=w372, element=T17."Intro", error in (no error)=w371) -> (queue out=w369:refnum<queue>, error out=w368:errorcluster)  [unwired: 1 in, 1 out]
        n193 = Enqueue Element(queue=w369, element=T17."Wait", error in (no error)=w368) -> (queue out=w367:refnum<queue>, error out=w366:errorcluster)  [unwired: 1 in, 1 out]
      }
      event "UlohaEDA": Value Change {
        n194 = event-data() -> ()  [unwired: 1 in, 6 out]
        n195 = Enqueue Element(queue=w380, element=T15."UlohaEDA", error in (no error)=w379) -> (queue out=w378:refnum<queue>, error out=w375:errorcluster)  [unwired: 1 in, 1 out]
        n196 = Enqueue Element(queue=w378, element=T15."Wait", error in (no error)=w375) -> (queue out=w377:refnum<queue>, error out=w376:errorcluster)  [unwired: 1 in, 1 out]
      }
      event "UlohaACC": Value Change {
        n197 = event-data() -> ()  [unwired: 1 in, 6 out]
        n198 = Enqueue Element(queue=w388, element=T15."UlohaACC", error in (no error)=w387) -> (queue out=w386:refnum<queue>, error out=w384:errorcluster)  [unwired: 1 in, 1 out]
        n199 = Enqueue Element(queue=w386, element=T15."Wait", error in (no error)=w384) -> (queue out=w385:refnum<queue>, error out=w383:errorcluster)  [unwired: 1 in, 1 out]
      }
      event "Playground": Value Change {
        n200 = event-data() -> ()  [unwired: 1 in, 6 out]
        n201 = Enqueue Element(queue=w396, element=T16."PlaygroundMeas", error in (no error)=w395) -> (queue out=w391:refnum<queue>, error out=w393:errorcluster)  [unwired: 1 in, 1 out]
        n202 = Enqueue Element(queue=w391, element=T16."Wait", error in (no error)=w393) -> (queue out=w390:refnum<queue>, error out=w392:errorcluster)  [unwired: 1 in, 1 out]
      }
      event "StopMeasure": Value Change {
        n203 = event-data() -> ()  [unwired: 1 in, 6 out]
        n204 = Enqueue Element(queue=w401, element=T16."PlaygroundMeas", error in (no error)=w399) -> (queue out=w400:refnum<queue>, error out=w398:errorcluster)  [unwired: 1 in, 1 out]
        n205 = property on="SyncStop" class="Bool (strict)"("Visible"=FALSE) -> ()  [unwired: 2 in, 2 out]
        n206 = Enqueue Element(queue=w400, element=enum16{"Wait", "Exit", "Measure"}."Wait", error in (no error)=w398) -> (queue out=w406:refnum<queue>, error out=w404:errorcluster)  [unwired: 1 in, 1 out]
        n207 = property on="SyncStop" class="Bool (strict)"(error in=w404, "Val(Sgnl)"=TRUE ("Value (Signaling)")) -> (error out=w403:errorcluster)  [unwired: 1 in, 1 out]
      }
      event "StopMeasureEKG": Value Change {
        n208 = event-data() -> ()  [unwired: 1 in, 6 out]
        n209 = Enqueue Element(queue=w417, element=T5."UlohaEKG", error in (no error)=w416) -> (queue out=w414:refnum<queue>, error out=w412:errorcluster)  [unwired: 1 in, 1 out]
        n210 = Enqueue Element(queue=w414, element=T5."Wait", error in (no error)=w412) -> (queue out=w413:refnum<queue>, error out=w410:errorcluster)  [unwired: 1 in, 1 out]
        n211 = property on="SyncStop 2" class="Bool (strict)"(error in=w410, "Value"=TRUE ("SyncStop 2")) -> (error out=w409:errorcluster)  [unwired: 1 in, 1 out]
      }
      event "StartMeasureEKG": Value Change {
        n212 = event-data() -> ()  [unwired: 1 in, 6 out]
        n213 = Enqueue Element(queue=w425, element=T5."UlohaEKG", error in (no error)=w424) -> (queue out=w423:refnum<queue>, error out=w421:errorcluster)  [unwired: 1 in, 1 out]
        n214 = Enqueue Element(queue=w423, element=T5."Measure", error in (no error)=w421) -> (queue out=w422:refnum<queue>, error out=w420:errorcluster)  [unwired: 1 in, 1 out]
      }
      event "StartMeasure": Value Change {
        n215 = event-data() -> ()  [unwired: 1 in, 6 out]
        n216 = Enqueue Element(queue=w430, element=T16."PlaygroundMeas", error in (no error)=w428) -> (queue out=w429:refnum<queue>, error out=w427:errorcluster)  [unwired: 1 in, 1 out]
        n217 = Enqueue Element(queue=w429, element=enum16{"Wait", "Exit", "Measure"}."Measure", error in (no error)=w427) -> (queue out=w433:refnum<queue>, error out=w432:errorcluster)  [unwired: 1 in, 1 out]
      }
      event "DeleteSignal": Value Change {
        n218 = event-data() -> ()  [unwired: 1 in, 6 out]
        n219 = Enqueue Element(queue=w441, element=T5."PlaygroundMeas", error in (no error)=w440) -> (queue out=w438:refnum<queue>, error out=w436:errorcluster)  [unwired: 1 in, 1 out]
        n220 = Enqueue Element(queue=w438, element=T5."DeleteSignal", error in (no error)=w436) -> (queue out=w437:refnum<queue>, error out=w435:errorcluster)  [unwired: 1 in, 1 out]
      }
      event "SendToFilter": Value Change {
        n221 = event-data() -> ()  [unwired: 1 in, 6 out]
        n222 = Enqueue Element(queue=w449, element=T18."PlaygroundFiltr", error in (no error)=w448) -> (queue out=w446:refnum<queue>, error out=w444:errorcluster)  [unwired: 1 in, 1 out]
        n223 = Enqueue Element(queue=w446, element=T18."Wait", error in (no error)=w444) -> (queue out=w445:refnum<queue>, error out=w443:errorcluster)  [unwired: 1 in, 1 out]
      }
      event "SaveFileButton": Value Change {
        n224 = event-data() -> ()  [unwired: 1 in, 6 out]
        n225 = Enqueue Element(queue=w454, element=T19."SaveFile", error in (no error)=w453) -> (queue out=w452:refnum<queue>, error out=w451:errorcluster)  [unwired: 1 in, 1 out]
      }
      event "Filtr": Value Change {
        n226 = event-data() -> ()  [unwired: 1 in, 6 out]
        n227 = Enqueue Element(queue=w462, element=T20."PlaygroundFiltr", error in (no error)=w459) -> (queue out=w461:refnum<queue>, error out=w458:errorcluster)  [unwired: 1 in, 1 out]
        n228 = Enqueue Element(queue=w461, element=T20."FilterSignal", error in (no error)=w458) -> (queue out=w460:refnum<queue>, error out=w457:errorcluster)  [unwired: 1 in, 1 out]
      }
      event "HintEKG": Value Change {
        n229 = event-data() -> ()  [unwired: 1 in, 6 out]
        n230 = Enqueue Element(queue=w470, element=T14."UlohaEKG", error in (no error)=w467) -> (queue out=w469:refnum<queue>, error out=w466:errorcluster)  [unwired: 1 in, 1 out]
        n231 = Enqueue Element(queue=w469, element=T14."HintEKG", error in (no error)=w466) -> (queue out=w468:refnum<queue>, error out=w465:errorcluster)  [unwired: 1 in, 1 out]
      }
    }
    n232 = Wait Until Next ms Multiple(millisecond multiple=u32 250) -> ()  [unwired: 1 out]
  }
  n233 = Release Queue(queue=w8, error in (no error)=w7) -> (error out=w4:errorcluster)  [unwired: 1 in, 2 out]
  n234 = Unregister For Events(event registration refnum=w5, error in=w4) -> (error out=w3:errorcluster)
  n235 = Destroy User Event(user event=w2, error in=w3) -> ()  [unwired: 1 out]
